vi "Initialize.vi"(8 "error in (no error)":errorcluster, 10 "Parameters in":refnum<class "Abstract Init Parameters.lvclass">, 11 "Abstract Consumer in":refnum<class "Abstract Consumer.lvclass">) -> (0 "error out":errorcluster, 3 "Abstract Consumer out":refnum<class "Abstract Consumer.lvclass">)   [LabVIEW 2027, in "Messaging.lvlib" / "Abstract Consumer.lvclass"]
uses:
  Abstract Consumer.lvclass
  Parameters/Abstract Init Parameters/Abstract Init Parameters.lvclass
  Abstract Consumer.lvclass/Abstract Consumer.ctl
  Messaging.lvlib
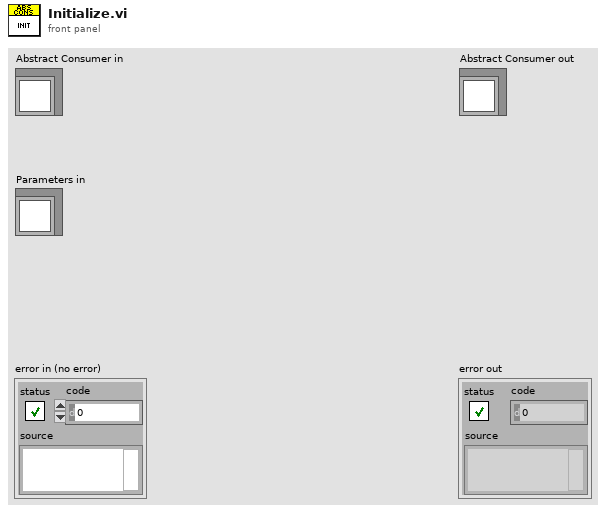
[diagram p1: front panel]
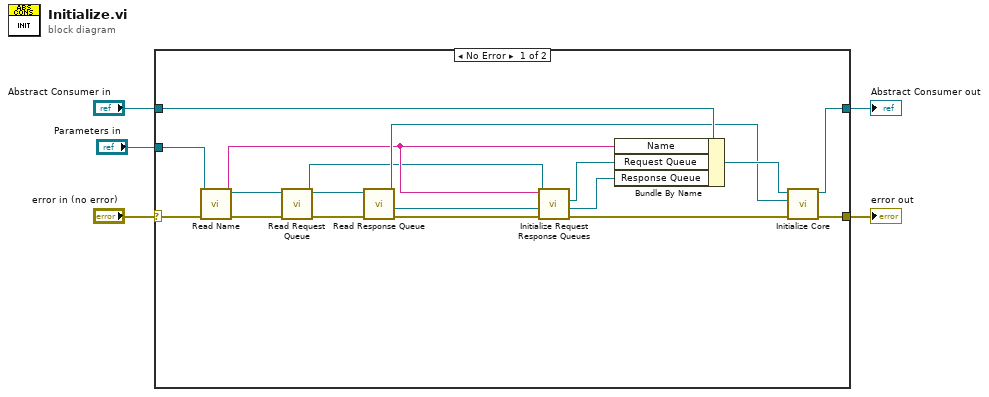
[diagram p0: block diagram]
diagram:
  n1 = case shown="No Error" "error in (no error)" {
    selector: "error in (no error)" -> [w11 w25]
    tunnel: [w19 w25] -> w4
    tunnel: [w17 w24] -> w2
    tunnel: "Abstract Consumer in" -> [w23 w24]
    tunnel: "Parameters in" -> [w12 _]
    frame No Error {
      n2 = call-dynamic "Read Name.vi"("error in (no error)"=w11, "Abstract Init Parameters in"=w12) -> ("error out"=w14:errorcluster, "Name"=w9:string, "Abstract Init Parameters out"=w16:refnum<class "Abstract Init Parameters.lvclass">)  [unwired: 7 in]
      n3 = call-dynamic "Read Request Queue.vi"("error in (no error)"=w14, "Abstract Init Parameters in"=w16) -> ("error out"=w13:errorcluster, "Message Queue Library.lvlib:Abstract Message Queue.lvclass"=w7:refnum<class "Abstract Message Queue.lvclass">, "Abstract Init Parameters out"=w15:refnum<class "Abstract Init Parameters.lvclass">)  [unwired: 7 in]
      n4 = call-dynamic "Read Response Queue.vi"("error in (no error)"=w13, "Abstract Init Parameters in"=w15) -> ("error out"=w8:errorcluster, "Message Queue Library.lvlib:Abstract Message Queue.lvclass"=w6:refnum<class "Abstract Message Queue.lvclass">, "Abstract Init Parameters out"=w10:refnum<class "Abstract Init Parameters.lvclass">)  [unwired: 7 in]
      n5 = call "Initialize Request Response Queues.vi"("error in (no error)"=w8, "Response Queue in"=w6, "Request Queue in"=w7, "Name"=w9) -> ("error out"=w20:errorcluster, "Response Queue out"=w21:refnum<class "Abstract Message Queue.lvclass">, "Request Queue out"=w22:refnum<class "Abstract Message Queue.lvclass">)  [unwired: 5 in]
      n6 = Bundle By Name(cluster=w23, "Name"=w9, "Request Queue"=w22, "Response Queue"=w21) -> (w18:refnum<class "Abstract Consumer.lvclass">)
      n7 = call-dynamic "Initialize Core.vi"("error in (no error)"=w20, "Parameters"=w10, "Abstract Consumer in"=w18) -> ("error out"=w19:errorcluster, "Abstract Consumer out"=w17:refnum<class "Abstract Consumer.lvclass">)  [unwired: 7 in]
    }
    frame Error {
    }
  }
  "error out" <- w4
  "Abstract Consumer out" <- w2
